vi "sin zivi.vi"() -> ()   [LabVIEW 2017]
uses:
  sin.vi
panel:
  out "波形图表":dbl(graph)
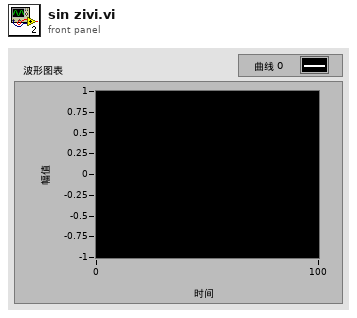
[diagram p1: front panel]
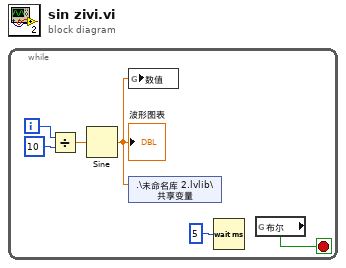
[diagram p0: block diagram]
diagram:
  n1 = while {
    i -> [w4]
    stop <- w6 stop-if-true
    n2 = Divide(x=w4, y=10) -> (x/y=w5:dbl)
    n3 = Sine(x=w5) -> (sin(x)=w3:dbl)
    "波形图表" <- w3
    n4 = global write "sin.vi" "数值"(w3) -> ()
    n5 = shared-variable ".\\未命名库 2.lvlib\\共享变量"(w3) -> ()  [unwired: 1 in, 1 out]
    n6 = Wait (ms)(milliseconds to wait=5) -> ()  [unwired: 1 out]
    n7 = global read "sin.vi" "布尔"() -> (w6:bool)
  }
